vi "HEXandASCIIConverter_XOR.vi"(10 "Boolean array2 in":bool[](array[boolean]), 11 "Boolean array1 in":bool[](array[boolean])) -> (1 "hex integer string":string, 2 "x .xor. y?":bool[](array[boolean]), 3 "number":u32, 4 "ASCII 格式輸出":string)   [LabVIEW 2019]
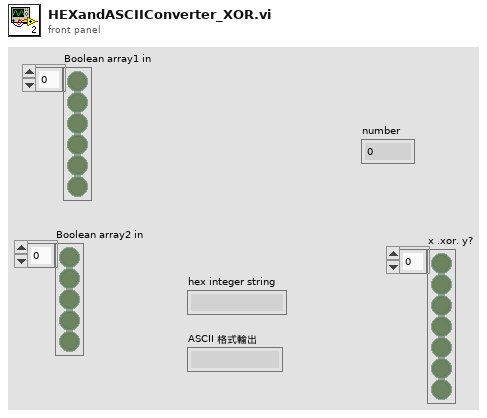
[diagram p1: front panel]
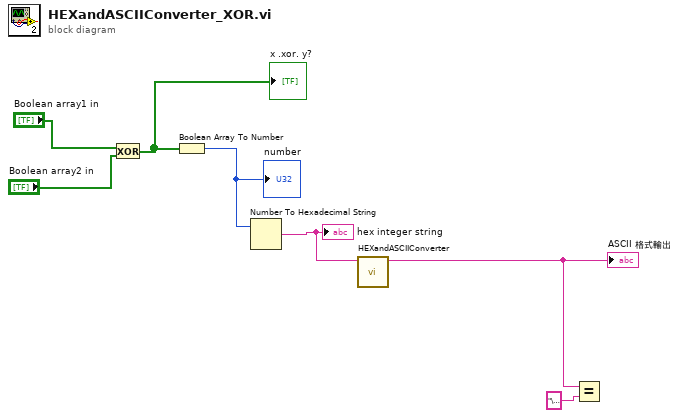
[diagram p0: block diagram]
diagram:
  n1 = Exclusive Or(1:"Boolean array2 in", 2:"Boolean array1 in") -> (0:w3:bool[])
  "x .xor. y?" <- w3
  n2 = Boolean Array To Number(Boolean array=w3) -> (number=w4:u32)
  "number" <- w4
  n3 = Number To Hexadecimal String(2:w4) -> (0:w6:string)  [unwired: 1 in]
  "hex integer string" <- w6
  n4 = call "HEXandASCIIConverter.vi"("HEX 格式輸入"=w6) -> ("ASCII 格式輸出"=w7:string)  [unwired: 8 in, 1 out]
  "ASCII 格式輸出" <- w7
  n5 = Equal?(x=w7, y="\u000f") -> ()  [unwired: 1 out]
